vi "Open Swerve Drive.vi"   [LabVIEW 2019]
uses:
  <vilib>/Rock Robotics/SystemInterfaces/AI/FPGA_AIChannel.ctl
types:
  T1 = typedef "FPGA_AIChannel.ctl" = enum8{"AI 0", "AI 1", "AI 2", "AI 3", "AI MXP 0", "AI MXP 1", "AI MXP 2", "AI MXP 3", "Invalid"}
  T2 = typedef "WPI_MotorControlDeviceRef.ctl" = cluster{"DeviceStatus":errorcluster, "Type":T3, "PWM":cluster{"PWM Channel":T4, "DeadBand":T5}, "CAN":cluster{"Device Number":u8, "SetOutput VI Ref":variant, "GetOutput VI Ref":variant, "Enable VI Ref":variant, "Disable VI Ref":variant, "Data":variant}, "Invert":bool, "DIO PWM":cluster{"PWM \"Enable\" Channel":T4, "DIOChannel":T6, "PWM Rate":dbl}}
  T3 = typedef "WPI_MotorControlType.ctl" = enum16{"PWM", "CAN", "DIO PWM"}
  T4 = typedef "FPGA_DIOPWMChannel.ctl" = enum8{"PWM 0", "PWM 1", "PWM 2", "PWM 3", "PWM 4", "PWM 5", "PWM 6", "PWM 7", "PWM 8", "PWM 9", "PWM MXP 0", "PWM MXP 1", "PWM MXP 2", "PWM MXP 3", "PWM MXP 4", "PWM MXP 5", "PWM MXP 6", "PWM MXP 7", "PWM MXP 8", "PWM MXP 9", "Invalid"}
  T5 = typedef "WPI_PWMDeadband.ctl" = cluster{"Name":string, "maxPositivePwm":i32, "minPositivePwm":i32, "centerPwm":i32, "maxNegativePwm":i32, "minNegativePwm":i32, "angularRange":u16}
  T6 = typedef "FPGA_DIOChannel.ctl" = enum8{"DIO 0", "DIO 1", "DIO 2", "DIO 3", "DIO 4", "DIO 5", "DIO 6", "DIO 7", "DIO 8", "DIO 9", "DIO MXP 0", "DIO MXP 1", "DIO MXP 2", "DIO MXP 3", "DIO MXP 4", "DIO MXP 5", "DIO MXP 6", "DIO MXP 7", "DIO MXP 8", "DIO MXP 9", "DIO MXP 10", "DIO MXP 11", "DIO MXP 12", "DIO MXP 13", "DIO MXP 14", "DIO MXP 15", "SPI Port CS1", "SPI Port CS2", "SPI Port CS3", "SPI Port MISO", "SPI Port MOSI", "Invalid"}
  T7 = typedef "WPI_AnalogChannelDevRef.ctl" = cluster{"DevStatus":errorcluster, "Analog Channel":T1}
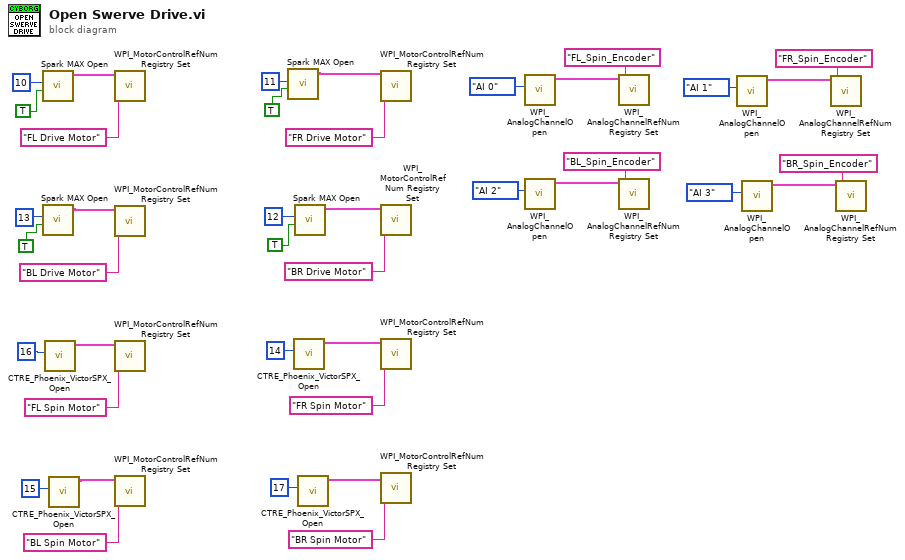
[diagram p0: block diagram]
diagram:
  n1 = call <vilib>:"Spark MAX Open.vi"("Invert"=TRUE, "Device Number"=u8 10) -> ("MotorControlDeviceRef"=w9:T2)  [unwired: 8 in, 1 out]
  n2 = call <vilib>:"Spark MAX Open.vi"("Invert"=TRUE, "Device Number"=u8 13) -> ("MotorControlDeviceRef"=w14:T2)  [unwired: 8 in, 1 out]
  n3 = call <vilib>:"CTRE_Phoenix_VictorSPX_Open.vi"("Device Number"=u8 16) -> ("CAN Talon SRX Ref"=w2:T2)  [unwired: 9 in, 1 out]
  n4 = call <vilib>:"CTRE_Phoenix_VictorSPX_Open.vi"("Device Number"=u8 15) -> ("CAN Talon SRX Ref"=w20:T2)  [unwired: 9 in, 1 out]
  n5 = call <vilib>:"WPI_MotorControlRefNum Registry Set.vi"("refnum name"="FL Drive Motor", "MotorControlDevRef"=w9) -> ()  [unwired: 8 in, 2 out]
  n6 = call <vilib>:"WPI_MotorControlRefNum Registry Set.vi"("refnum name"="BL Drive Motor", "MotorControlDevRef"=w14) -> ()  [unwired: 8 in, 2 out]
  n7 = call <vilib>:"WPI_MotorControlRefNum Registry Set.vi"("refnum name"="FL Spin Motor", "MotorControlDevRef"=w2) -> ()  [unwired: 8 in, 2 out]
  n8 = call <vilib>:"WPI_MotorControlRefNum Registry Set.vi"("refnum name"="BL Spin Motor", "MotorControlDevRef"=w20) -> ()  [unwired: 8 in, 2 out]
  n9 = call <vilib>:"Spark MAX Open.vi"("Invert"=TRUE, "Device Number"=u8 11) -> ("MotorControlDeviceRef"=w7:T2)  [unwired: 8 in, 1 out]
  n10 = call <vilib>:"CTRE_Phoenix_VictorSPX_Open.vi"("Device Number"=u8 14) -> ("CAN Talon SRX Ref"=w19:T2)  [unwired: 9 in, 1 out]
  n11 = call <vilib>:"Spark MAX Open.vi"("Invert"=TRUE, "Device Number"=u8 12) -> ("MotorControlDeviceRef"=w4:T2)  [unwired: 8 in, 1 out]
  n12 = call <vilib>:"CTRE_Phoenix_VictorSPX_Open.vi"("Device Number"=u8 17) -> ("CAN Talon SRX Ref"=w18:T2)  [unwired: 9 in, 1 out]
  n13 = call <vilib>:"WPI_MotorControlRefNum Registry Set.vi"("refnum name"="FR Drive Motor", "MotorControlDevRef"=w7) -> ()  [unwired: 8 in, 2 out]
  n14 = call <vilib>:"WPI_MotorControlRefNum Registry Set.vi"("refnum name"="BR Drive Motor", "MotorControlDevRef"=w4) -> ()  [unwired: 8 in, 2 out]
  n15 = call <vilib>:"WPI_MotorControlRefNum Registry Set.vi"("refnum name"="FR Spin Motor", "MotorControlDevRef"=w19) -> ()  [unwired: 8 in, 2 out]
  n16 = call <vilib>:"WPI_MotorControlRefNum Registry Set.vi"("refnum name"="BR Spin Motor", "MotorControlDevRef"=w18) -> ()  [unwired: 8 in, 2 out]
  n17 = call <vilib>:"WPI_AnalogChannelOpen.vi"("Analog Channel"=FPGA_AIChannel."AI 0") -> ("AIDeviceRef"=w28:T7)  [unwired: 9 in, 1 out]
  n18 = call <vilib>:"WPI_AnalogChannelOpen.vi"("Analog Channel"=FPGA_AIChannel."AI 2") -> ("AIDeviceRef"=w31:T7)  [unwired: 9 in, 1 out]
  n19 = call <vilib>:"WPI_AnalogChannelRefNum Registry Set.vi"("refnum name"="FL_Spin_Encoder", "AIDeviceRef"=w28) -> ()  [unwired: 8 in, 2 out]
  n20 = call <vilib>:"WPI_AnalogChannelRefNum Registry Set.vi"("refnum name"="BL_Spin_Encoder", "AIDeviceRef"=w31) -> ()  [unwired: 8 in, 2 out]
  n21 = call <vilib>:"WPI_AnalogChannelOpen.vi"("Analog Channel"=FPGA_AIChannel."AI 1") -> ("AIDeviceRef"=w25:T7)  [unwired: 9 in, 1 out]
  n22 = call <vilib>:"WPI_AnalogChannelOpen.vi"("Analog Channel"=FPGA_AIChannel."AI 3") -> ("AIDeviceRef"=w22:T7)  [unwired: 9 in, 1 out]
  n23 = call <vilib>:"WPI_AnalogChannelRefNum Registry Set.vi"("refnum name"="FR_Spin_Encoder", "AIDeviceRef"=w25) -> ()  [unwired: 8 in, 2 out]
  n24 = call <vilib>:"WPI_AnalogChannelRefNum Registry Set.vi"("refnum name"="BR_Spin_Encoder", "AIDeviceRef"=w22) -> ()  [unwired: 8 in, 2 out]
